vi "Font Global.vi"() -> ()   [LabVIEW 2016, in "Code String.lvclass"]
doc: "Global variable to hold font parameters (name, size, etc.)."
uses:
  Code String.lvclass
panel:
  in  "Font Size":u32=14
  out "Font":string="Consolas"
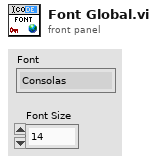
[diagram p1: front panel]
diagram:
